vi "KnowPosition.vi"() -> ()   [LabVIEW 2018]
uses:
  outputs.vi
  sensors.vi
  refnums.vi
panel:
  out "Robot Position":cluster{dbl[], dbl[]}(graph)
  in  "Reset Positon":bool
  out "Heading (deg)":dbl format="%#_13g"
  out "Y Position (in)":dbl
  out "X Position (in)":dbl
  in  "Plot Data":bool
  out "Drive Encoder Velocities":cluster{dbl, dbl}
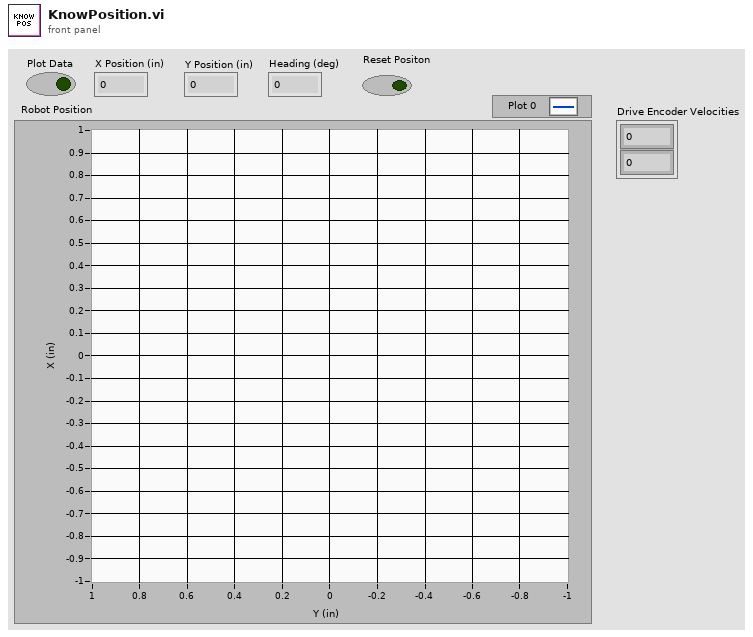
[diagram p1: front panel]
types:
  T1 = typedef "WPI_MotorControlDeviceRef.ctl" = cluster{"DeviceStatus":errorcluster, "Type":T2, "PWM":cluster{"PWM Channel":T3, "DeadBand":T4}, "CAN":cluster{"Device Number":u8, "SetOutput VI Ref":variant, "GetOutput VI Ref":variant, "Enable VI Ref":variant, "Disable VI Ref":variant, "Data":variant}, "Invert":bool, "DIO PWM":cluster{"PWM \"Enable\" Channel":T3, "DIOChannel":T5, "PWM Rate":dbl}}
  T2 = typedef "WPI_MotorControlType.ctl" = enum16{"PWM", "CAN", "DIO PWM"}
  T3 = typedef "FPGA_DIOPWMChannel.ctl" = enum8{"PWM 0", "PWM 1", "PWM 2", "PWM 3", "PWM 4", "PWM 5", "PWM 6", "PWM 7", "PWM 8", "PWM 9", "PWM MXP 0", "PWM MXP 1", "PWM MXP 2", "PWM MXP 3", "PWM MXP 4", "PWM MXP 5", "PWM MXP 6", "PWM MXP 7", "PWM MXP 8", "PWM MXP 9", "Invalid"}
  T4 = typedef "WPI_PWMDeadband.ctl" = cluster{"Name":string, "maxPositivePwm":i32, "minPositivePwm":i32, "centerPwm":i32, "maxNegativePwm":i32, "minNegativePwm":i32, "angularRange":u16}
  T5 = typedef "FPGA_DIOChannel.ctl" = enum8{"DIO 0", "DIO 1", "DIO 2", "DIO 3", "DIO 4", "DIO 5", "DIO 6", "DIO 7", "DIO 8", "DIO 9", "DIO MXP 0", "DIO MXP 1", "DIO MXP 2", "DIO MXP 3", "DIO MXP 4", "DIO MXP 5", "DIO MXP 6", "DIO MXP 7", "DIO MXP 8", "DIO MXP 9", "DIO MXP 10", "DIO MXP 11", "DIO MXP 12", "DIO MXP 13", "DIO MXP 14", "DIO MXP 15", "SPI Port CS1", "SPI Port CS2", "SPI Port CS3", "SPI Port MISO", "SPI Port MOSI", "Invalid"}
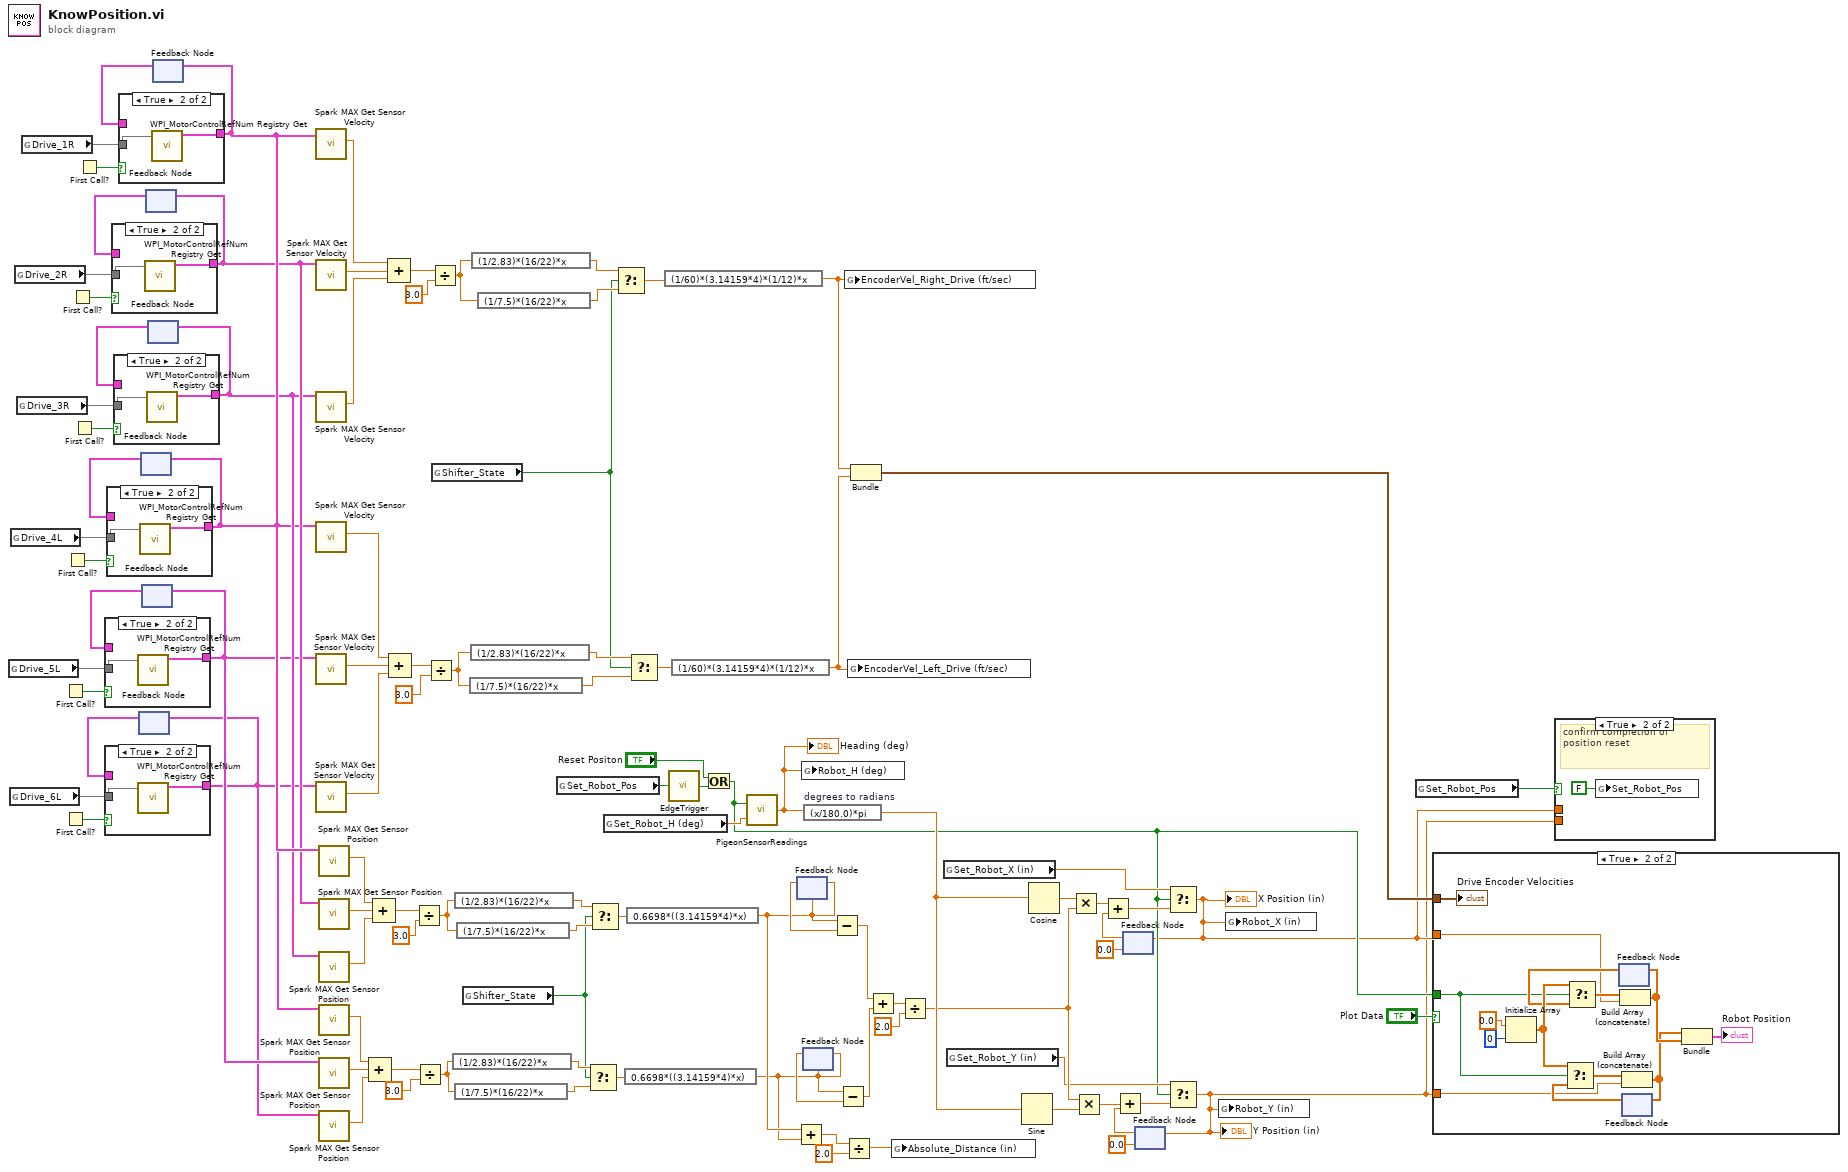
[diagram p0: block diagram]
diagram:
  n1 = global read "refnums.vi" "Drive_5L"() -> (w31)
  n2 = global read "refnums.vi" "Drive_6L"() -> (w27)
  n3 = global read "refnums.vi" "Drive_4L"() -> (w38)
  n4 = global read "refnums.vi" "Drive_2R"() -> (w44)
  n5 = global read "refnums.vi" "Drive_3R"() -> (w41)
  n6 = global read "refnums.vi" "Drive_1R"() -> (w47)
  n7 = First Call?() -> (First Call?: T/F=w33:bool)
  n8 = First Call?() -> (First Call?: T/F=w29:bool)
  n9 = First Call?() -> (First Call?: T/F=w40:bool)
  n10 = First Call?() -> (First Call?: T/F=w46:bool)
  n11 = First Call?() -> (First Call?: T/F=w43:bool)
  n12 = First Call?() -> (First Call?: T/F=w49:bool)
  n13 = feedback #1() -> (w28:T1)  [unwired: 1 in]
  n14 = case shown="True" w29 {
    tunnel: [w101 w102] -> w26
    tunnel: w28 -> [w101 _]
    tunnel: w27 -> [_ w103]
    frame False {
    }
    frame True {
      n15 = call <vilib>:"WPI_MotorControlRefNum Registry Get.vi"("refnum name"=w103) -> ("MotorControlDevRef"=w102:T1)  [unwired: 9 in, 1 out]
    }
  }
  n16 = feedback-in #1(w26) -> ()
  n17 = feedback #2() -> (w39:T1)  [unwired: 1 in]
  n18 = case shown="True" w40 {
    tunnel: [w104 w105] -> w34
    tunnel: w39 -> [w104 _]
    tunnel: w38 -> [_ w106]
    frame False {
    }
    frame True {
      n19 = call <vilib>:"WPI_MotorControlRefNum Registry Get.vi"("refnum name"=w106) -> ("MotorControlDevRef"=w105:T1)  [unwired: 9 in, 1 out]
    }
  }
  n20 = feedback-in #2(w34) -> ()
  n21 = feedback #3() -> (w32:T1)  [unwired: 1 in]
  n22 = case shown="True" w33 {
    tunnel: [w107 w108] -> w30
    tunnel: w32 -> [w107 _]
    tunnel: w31 -> [_ w109]
    frame False {
    }
    frame True {
      n23 = call <vilib>:"WPI_MotorControlRefNum Registry Get.vi"("refnum name"=w109) -> ("MotorControlDevRef"=w108:T1)  [unwired: 9 in, 1 out]
    }
  }
  n24 = feedback-in #3(w30) -> ()
  n25 = feedback #4() -> (w45:T1)  [unwired: 1 in]
  n26 = case shown="True" w46 {
    tunnel: [w110 w111] -> w36
    tunnel: w45 -> [w110 _]
    tunnel: w44 -> [_ w112]
    frame False {
    }
    frame True {
      n27 = call <vilib>:"WPI_MotorControlRefNum Registry Get.vi"("refnum name"=w112) -> ("MotorControlDevRef"=w111:T1)  [unwired: 9 in, 1 out]
    }
  }
  n28 = feedback-in #4(w36) -> ()
  n29 = feedback #5() -> (w42:T1)  [unwired: 1 in]
  n30 = case shown="True" w43 {
    tunnel: [w113 w114] -> w35
    tunnel: w42 -> [w113 _]
    tunnel: w41 -> [_ w115]
    frame False {
    }
    frame True {
      n31 = call <vilib>:"WPI_MotorControlRefNum Registry Get.vi"("refnum name"=w115) -> ("MotorControlDevRef"=w114:T1)  [unwired: 9 in, 1 out]
    }
  }
  n32 = feedback-in #5(w35) -> ()
  n33 = feedback #6() -> (w48:T1)  [unwired: 1 in]
  n34 = case shown="True" w49 {
    tunnel: [w116 w117] -> w37
    tunnel: w48 -> [w116 _]
    tunnel: w47 -> [_ w118]
    frame False {
    }
    frame True {
      n35 = call <vilib>:"WPI_MotorControlRefNum Registry Get.vi"("refnum name"=w118) -> ("MotorControlDevRef"=w117:T1)  [unwired: 9 in, 1 out]
    }
  }
  n36 = feedback-in #6(w37) -> ()
  n37 = call <vilib>:"Spark MAX Get Sensor Velocity.vi"("MotorControlDevRef in"=w37) -> ("Sensor Velocity"=w100:dbl)  [unwired: 7 in, 3 out]
  n38 = call <vilib>:"Spark MAX Get Sensor Velocity.vi"("MotorControlDevRef in"=w36) -> ("Sensor Velocity"=w99:dbl)  [unwired: 7 in, 3 out]
  n39 = call <vilib>:"Spark MAX Get Sensor Velocity.vi"("MotorControlDevRef in"=w35) -> ("Sensor Velocity"=w98:dbl)  [unwired: 7 in, 3 out]
  n40 = call <vilib>:"Spark MAX Get Sensor Velocity.vi"("MotorControlDevRef in"=w34) -> ("Sensor Velocity"=w97:dbl)  [unwired: 7 in, 3 out]
  n41 = call <vilib>:"Spark MAX Get Sensor Velocity.vi"("MotorControlDevRef in"=w30) -> ("Sensor Velocity"=w96:dbl)  [unwired: 7 in, 3 out]
  n42 = call <vilib>:"Spark MAX Get Sensor Velocity.vi"("MotorControlDevRef in"=w26) -> ("Sensor Velocity"=w95:dbl)  [unwired: 7 in, 3 out]
  n43 = call <vilib>:"Spark MAX Get Sensor Position.vi"("MotorControlDevRef in"=w37) -> ("Sensor Position"=w80:dbl)  [unwired: 7 in, 3 out]
  n44 = call <vilib>:"Spark MAX Get Sensor Position.vi"("MotorControlDevRef in"=w36) -> ("Sensor Position"=w79:dbl)  [unwired: 7 in, 3 out]
  n45 = call <vilib>:"Spark MAX Get Sensor Position.vi"("MotorControlDevRef in"=w35) -> ("Sensor Position"=w78:dbl)  [unwired: 7 in, 3 out]
  n46 = call <vilib>:"Spark MAX Get Sensor Position.vi"("MotorControlDevRef in"=w34) -> ("Sensor Position"=w73:dbl)  [unwired: 7 in, 3 out]
  n47 = call <vilib>:"Spark MAX Get Sensor Position.vi"("MotorControlDevRef in"=w30) -> ("Sensor Position"=w72:dbl)  [unwired: 7 in, 3 out]
  n48 = call <vilib>:"Spark MAX Get Sensor Position.vi"("MotorControlDevRef in"=w26) -> ("Sensor Position"=w71:dbl)  [unwired: 7 in, 3 out]
  n49 = Compound Arithmetic op=ADD(w73, w72, w71) -> (w75:dbl)
  n50 = Compound Arithmetic op=ADD(w80, w79, w78) -> (w77:dbl)
  n51 = Compound Arithmetic op=ADD(w100, w99, w98) -> (w92:dbl)
  n52 = Compound Arithmetic op=ADD(w97, w96, w95) -> (w91:dbl)
  n53 = Divide(x=w77, y=3.0) -> (x/y=w20:dbl)
  n54 = Divide(x=w75, y=3.0) -> (x/y=w16:dbl)
  n55 = Divide(x=w91, y=3.0) -> (x/y=w90:dbl)
  n56 = Divide(x=w92, y=3.0) -> (x/y=w89:dbl)
  n57 = global read "outputs.vi" "Shifter_State"() -> (w52:bool)
  n58 = expression code="(1/2.83)*(16/22)*x"(w16) -> (w15:dbl)
  n59 = expression code="(1/2.83)*(16/22)*x"(w20) -> (w59:dbl)
  n60 = expression code="(1/7.5)*(16/22)*x"(w16) -> (w18:dbl)
  n61 = expression code="(1/7.5)*(16/22)*x"(w20) -> (w58:dbl)
  n62 = global read "outputs.vi" "Shifter_State"() -> (w12:bool)
  n63 = expression code="(1/7.5)*(16/22)*x"(w90) -> (w85:dbl)
  n64 = expression code="(1/2.83)*(16/22)*x"(w90) -> (w86:dbl)
  n65 = expression code="(1/2.83)*(16/22)*x"(w89) -> (w88:dbl)
  n66 = expression code="(1/7.5)*(16/22)*x"(w89) -> (w87:dbl)
  n67 = global read "sensors.vi" "Set_Robot_Pos"() -> (w8:bool)
  n68 = Select(t=w15, s=w12, f=w18) -> (s? t:f=w17:dbl)
  n69 = Select(t=w59, s=w12, f=w58) -> (s? t:f=w53:dbl)
  n70 = global read "sensors.vi" "Set_Robot_H (deg)"() -> (w9:dbl)
  n71 = Select(t=w88, s=w52, f=w87) -> (s? t:f=w84:dbl)
  n72 = expression code="0.6698*((3.14159*4)*x)"(w17) -> (w14:dbl)
  n73 = expression code="0.6698*((3.14159*4)*x)"(w53) -> (w19:dbl)
  n74 = Select(t=w86, s=w52, f=w85) -> (s? t:f=w83:dbl)
  n75 = expression code="(1/60)*(3.14159*4)*(1/12)*x"(w84) -> (w50:dbl)
  n76 = call "EdgeTrigger.vi"("Input Signal"=w8) -> ("All Edge Trigger"=w7:bool)  [unwired: 2 out]
  n77 = expression code="(1/60)*(3.14159*4)*(1/12)*x"(w83) -> (w51:dbl)
  n78 = Or(x="Reset Positon", y=w7) -> (x .or. y?=w5:bool)
  n79 = call "PigeonSensorReadings.vi"("Reset Yaw (deg)"=w9, "Reset Yaw"=w5) -> ("Yaw (deg)"=w1:dbl)
  "Heading (deg)" <- w1
  n80 = Add(x=w19, y=w14) -> (x+y=w23:dbl)
  n81 = feedback-in #7(w19) -> ()
  n82 = feedback #7(w19) -> (w57:dbl)
  n83 = global write "sensors.vi" "Robot_H (deg)"(w1) -> ()
  n84 = feedback #8(w14) -> (w56:dbl)
  n85 = feedback-in #8(w14) -> ()
  n86 = expression code="(x/180.0)*pi" "degrees to radians"(w1) -> (w60:dbl)
  n87 = Subtract(x=w19, y=w57) -> (x-y=w25:dbl)
  n88 = Subtract(x=w14, y=w56) -> (x-y=w24:dbl)
  n89 = Divide(x=w23, y=2.0) -> (x/y=w13:dbl)
  n90 = global write "sensors.vi" "EncoderVel_Right_Drive (ft/sec)"(w50) -> ()
  n91 = global write "sensors.vi" "EncoderVel_Left_Drive (ft/sec)"(w51) -> ()
  n92 = Bundle(w50, w51) -> (w81:cluster{dbl, dbl})  [unwired: 1 in]
  n93 = Add(x=w25, y=w24) -> (x+y=w70:dbl)
  n94 = global write "sensors.vi" "Absolute_Distance (in)"(w13) -> ()
  n95 = Divide(x=w70, y=2.0) -> (x/y=w21:dbl)
  n96 = global read "sensors.vi" "Set_Robot_X (in)"() -> (w11:dbl)
  n97 = global read "sensors.vi" "Set_Robot_Y (in)"() -> (w10:dbl)
  n98 = Sine(x=w60) -> (sin(x)=w67:dbl)
  n99 = Cosine(x=w60) -> (cos(x)=w68:dbl)
  n100 = Multiply(x=w68, y=w21) -> (x*y=w66:dbl)
  n101 = Multiply(x=w21, y=w67) -> (x*y=w64:dbl)
  n102 = feedback #9(0.0) -> (w65:dbl)
  n103 = Add(x=w66, y=w65) -> (x+y=w54:dbl)
  n104 = feedback #10(0.0) -> (w63:dbl)
  n105 = Add(x=w64, y=w63) -> (x+y=w55:dbl)
  n106 = Select(t=w11, s=w5, f=w54) -> (s? t:f=w3:dbl)
  "X Position (in)" <- w3
  n107 = feedback-in #9(w3) -> ()
  n108 = Select(t=w10, s=w5, f=w55) -> (s? t:f=w2:dbl)
  "Y Position (in)" <- w2
  n109 = feedback-in #10(w2) -> ()
  n110 = global write "sensors.vi" "Robot_Y (in)"(w2) -> ()
  n111 = global write "sensors.vi" "Robot_X (in)"(w3) -> ()
  n112 = global read "sensors.vi" "Set_Robot_Pos"() -> (w4:bool)
  n113 = case shown="True" "Plot Data" {
    tunnel: w81 -> [_ w132]
    tunnel: w5 -> [_ w119]
    tunnel: w3 -> [_ w122]
    tunnel: w2 -> [_ w121]
    frame False {
    }
    frame True {
      n114 = Initialize Array(0.0 ("element"), 0 ("dimension size")) -> (w131:dbl[])
      n115 = feedback #11() -> (w127:dbl[])  [unwired: 1 in]
      n116 = Select(t=w131, s=w119, f=w127) -> (s? t:f=w128:dbl[])
      n117 = Build Array (concatenate)(w128, w122) -> (w126:dbl[])
      n118 = feedback-in #11(w126) -> ()
      n119 = feedback #12() -> (w129:dbl[])  [unwired: 1 in]
      n120 = Select(t=w131, s=w119, f=w129) -> (s? t:f=w130:dbl[])
      n121 = Build Array (concatenate)(w130, w121) -> (w125:dbl[])
      n122 = feedback-in #12(w125) -> ()
      n123 = Bundle(w125, w126) -> (→"Robot Position":cluster{dbl[], dbl[]})  [unwired: 1 in]
      "Drive Encoder Velocities" <- w132
    }
  }
  n124 = case shown="True" w4 {
    tunnel: w3 -> [_ _]
    tunnel: w2 -> [_ _]
    frame False {
    }
    frame True {
      # "confirm completion of position reset"
      n125 = global write "sensors.vi" "Set_Robot_Pos"(FALSE ("Set_Robot_Pos")) -> ()
    }
  }
